vi "BRig_RT__Case_Exp__storeData__endExp__v5__p3__v2.vi"(0 "input_prevStorage":bool, 7 "input_True":bool=TRUE, 9 "input_dataAnalog":u16[][](array[numeric]), 12 "input_count":i32) -> (8 "output_True":bool)   [LabVIEW 2014]
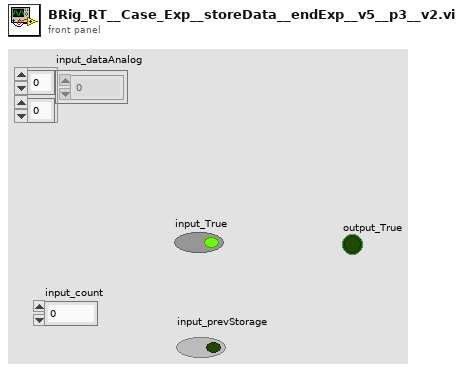
[diagram p1: front panel]
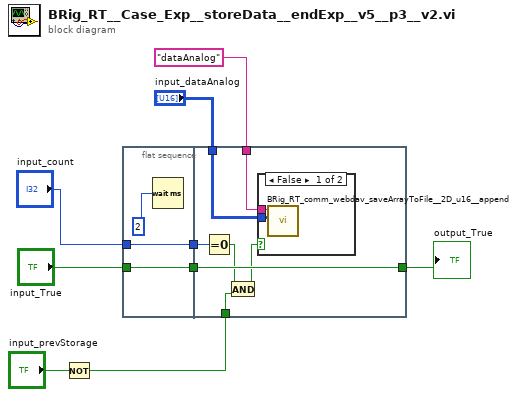
[diagram p0: block diagram]
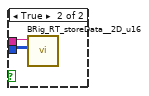
[diagram p2: hidden frame]
diagram:
  n1 = Not(x="input_prevStorage") -> (.not. x?=w1:bool)
  n2 = flat-sequence {
    tunnel: [w12] -> w7
    tunnel: "input_True" -> [w12]
    tunnel: "input_count" -> [w11]
    tunnel: [w11] -> w3
    tunnel: "input_dataAnalog" -> [w17]
    tunnel: "dataAnalog" ("input_filename") -> [w19]
    tunnel: w7 -> [w18]
    tunnel: [w18] -> w6
    tunnel: w3 -> [w16]
    tunnel: w1 -> [w13]
    frame #0 {
      n3 = Wait (ms)(milliseconds to wait=u32 2) -> ()  [unwired: 1 out]
    }
    frame #1 {
      n4 = Equal To 0?(x=w16) -> (x = 0?=w15:bool)
      n5 = And(x=w15, y=w13) -> (x .and. y?=w14:bool)
      n6 = case shown="False" w14 {
        tunnel: w19 -> [w21 w23]
        tunnel: w17 -> [w20 w22]
        frame False {
          n7 = call "BRig_RT_comm_webdav_saveArrayToFile__2D_u16__append.vi"("Array"=w20, "input_filename"=w21) -> ()  [unwired: 10 in]
        }
        frame True {
          n8 = call "BRig_RT_storeData__2D_u16.vi"("Array"=w22, "input_filename"=w23) -> ()  [unwired: 10 in]
        }
      }
    }
  }
  "output_True" <- w6
